vi "SubVI.vi"(11 "Data Value Reference in":refnum<data-value>) -> (3 "Data Value Reference out":refnum<data-value>)   [LabVIEW 2015]
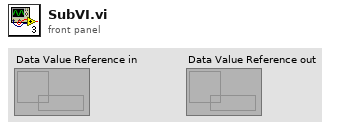
[diagram p1: front panel]
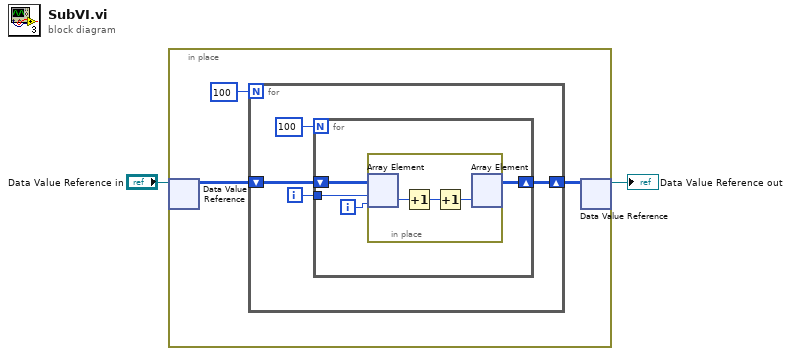
[diagram p0: block diagram]
diagram:
  n1 = in-place {
    n2 = in-place-dvr #1("Data Value Reference in") -> (w5:i32[][])  [unwired: 1 out]
    n3 = for {
      N: 100 ("dimension size") -> [_]
      shift-right: [w8] -> w3
      shift-left: w5 -> [w9]
      i -> [w6]
      n4 = for {
        N: 100 ("dimension size") -> [_]
        tunnel: w6 -> [w11]
        shift-right: [w12] -> w8
        shift-left: w9 -> [w13]
        i -> [w10]
        n5 = in-place {
          n6 = in-place-array #2(w13, w11, w10) -> (w16:i32)
          n7 = Increment(x=w16) -> (x+1=w15:i32)
          n8 = Increment(x=w15) -> (x+1=w14:i32)
          n9 = in-place-array #2(w14) -> (w12:i32[][])  [unwired: 2 out]
        }
      }
    }
    n10 = in-place-dvr #1(w3) -> (→"Data Value Reference out":refnum<data-value>)  [unwired: 1 out]
  }
